vi "myDAQ Optical Theremin.vi"() -> ()   [LabVIEW 2012]
uses:
  <vilib>/Analysis/baseanly.llb/Mean (DBL).vi
  <vilib>/Analysis/NI_AALBase.lvlib
panel:
  in  "切换开关":bool
  out "Gain":dbl(graph)=0.030011962890625
  out "音调输入幅值":dbl(knob) scale=0.0..10.0 scale format="%#_6p"
  out "音量输入幅值":dbl(knob) scale=0.0..10.0 scale format="%#_6p"
  in  "最小值":dbl(slide) scale=0.0..10.0
  in  "最大值":dbl(slide)=10.0 scale=0.0..10.0
  in  "最小值":dbl(slide) scale=0.0..10.0
  in  "最大值":dbl(slide)=10.0 scale=0.0..10.0
  in  "最大频率":dbl(knob)=880.0 scale=0.0..20000.0 scale format="%#_6p"
  in  "最小频率":dbl(knob)=440.0 scale=0.0..20000.0 scale format="%#_6p"
  in  "stop":bool
  out "Pitch":dbl(graph)=451.48833984375
  # "基于myDAQ的特雷门琴设计"
  # "音调控制"
  # "音量控制"
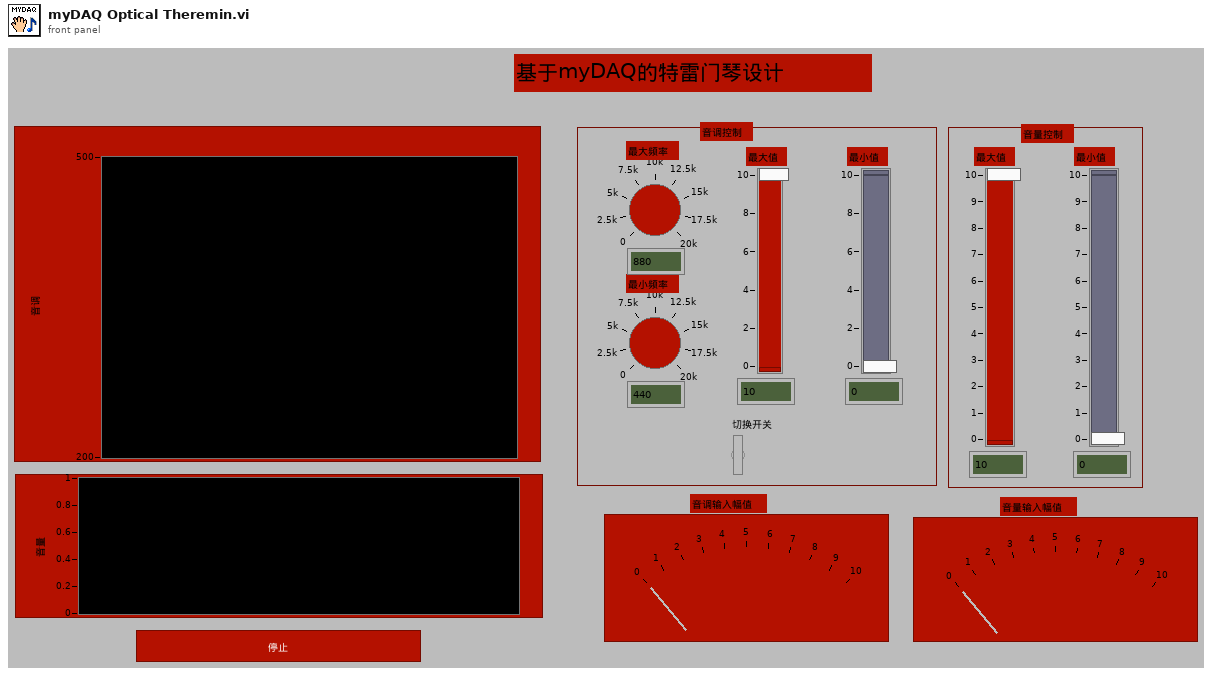
[diagram p1: front panel]
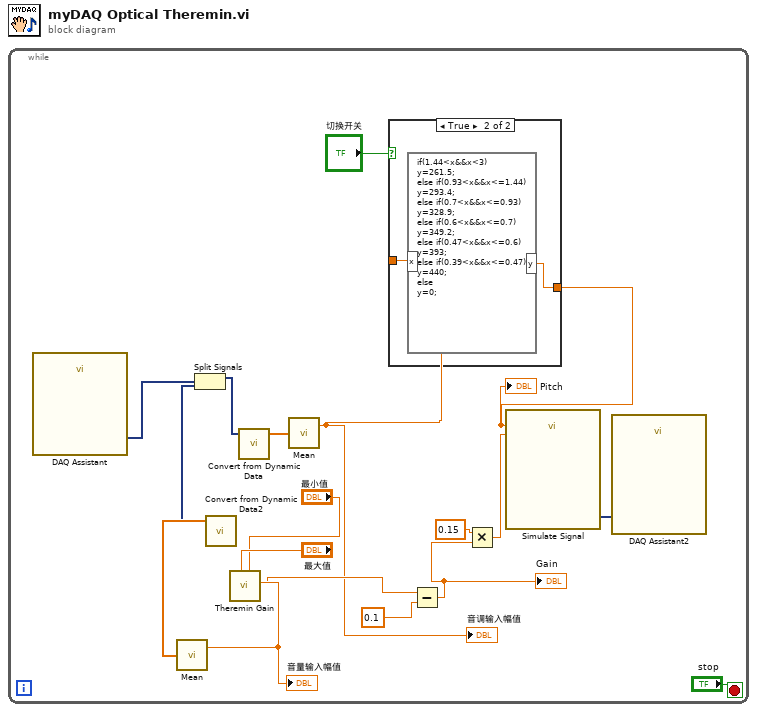
[diagram p0: block diagram]
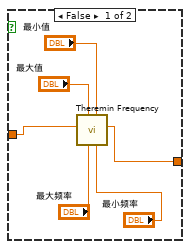
[diagram p2: hidden frame]
diagram:
  n1 = while {
    stop <- "stop" stop-if-true
    n2 = call "DAQ Assistant"() -> ("data"=w8:dynamicdata)  [unwired: 17 in, 2 out]
    n3 = Split Signals(w8) -> (w15:dynamicdata, w13:dynamicdata)  [unwired: 2 in]
    n4 = call "Convert from Dynamic Data2"("Dynamic Data Type"=w13) -> ("Array"=w14:dbl[])  [unwired: 3 in]
    n5 = call-poly <vilib>:"Mean.vi"("X"=w14) -> ("mean"=w7:dbl)  [unwired: 1 out]
    "音量输入幅值" <- w7
    n6 = call "Theremin Gain.vi"("Min Amp"="最小值", "Max Amp"="最大值", "Input Amp"=w7) -> ("Output Gain"=w6:dbl)  [unwired: 8 in]
    n7 = call "Convert from Dynamic Data"("Dynamic Data Type"=w15) -> ("Array"=w16:dbl[])  [unwired: 3 in]
    n8 = call-poly <vilib>:"Mean.vi"("X"=w16) -> ("mean"=w1:dbl)  [unwired: 1 out]
    "音调输入幅值" <- w1
    n9 = case shown="True" "切换开关" {
      tunnel: [w23 w26] -> w3
      tunnel: w1 -> [w19 w25]
      frame False {
        n10 = call "Theremin Frequency.vi"("Min Freq"="最小频率", "Min Amp"="最小值", "Max Freq"="最大频率", "Max Amp"="最大值", "Input Amp"=w19) -> ("Output Freq"=w23:dbl)  [unwired: 6 in]
      }
      frame True {
        n11 = formula code="if(1.44<x&&x<3)\ny=261.5;\nelse if(0.93<x&&x<=1.44)\ny=293.4;\nelse if(0.7<x&&x<=0.93)\ny=328.9;\nelse if(0.6<x&&x<=0.7)\ny=349.2;\nelse if(0.47<x&&x<=0.6)\ny=393;\nelse if(0.39<x&&x<=0.47)\ny=440;\nelse\ny=0;"("x"=w25) -> ("y"=w26:dbl)
      }
    }
    "Pitch" <- w3
    n12 = Subtract(x=w6, y=0.1) -> (x-y=w4:dbl)
    "Gain" <- w4
    n13 = Multiply(x=0.15, y=w4) -> (x*y=w9:dbl)
    n14 = call "Simulate Signal"("Frequency"=w3, "Amplitude"=w9) -> ("Sine"=w17:dynamicdata)  [unwired: 12 in, 1 out]
    n15 = call "DAQ Assistant2"("data"=w17) -> ()  [unwired: 16 in, 3 out]
  }
